vi "API_GetWindowhWnd by private Property.vi"(8 "错误输入（无错误）":errorcluster, 11 "VI引用句柄":refnum<vi>) -> (0 "错误输出":errorcluster, 2 "Front Panel Window:Native Window":u64, 3 "引用输出":refnum<vi>)   [LabVIEW 2011, in "API.lvlib"]
uses:
  API.lvlib
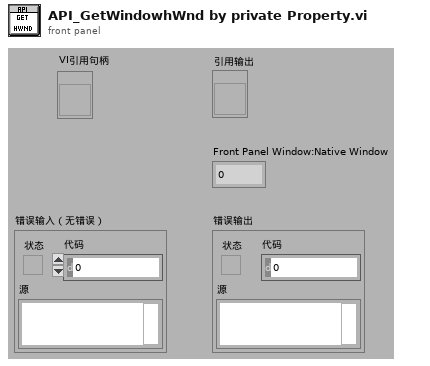
[diagram p1: front panel]
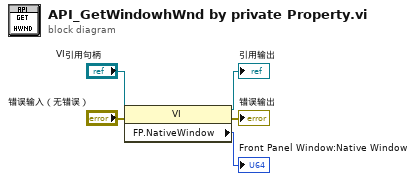
[diagram p0: block diagram]
diagram:
  n1 = property class="VI"(reference="VI引用句柄", error in="错误输入（无错误）") -> (reference out=→"引用输出":refnum<vi>, error out=→"错误输出":errorcluster, "FP.NativeWindow"=→"Front Panel Window:Native Window":u64)
